vi "AP_2_launcher.vi"() -> ()   [LabVIEW 2023]
panel:
  in  "Cold head control launch":bool
  in  "Delay Control Launch":bool
  in  "Stop":bool
  in  "PDS Acquisition Launch Button":bool
  in  "PES Acquisition Launch Button":bool
  in  "Oscilloscope Launch Button":bool
  # "AP-2 Software Launcher"
  # "Welcome to the AP-2 software suite! Please seclect the software you wish to use."
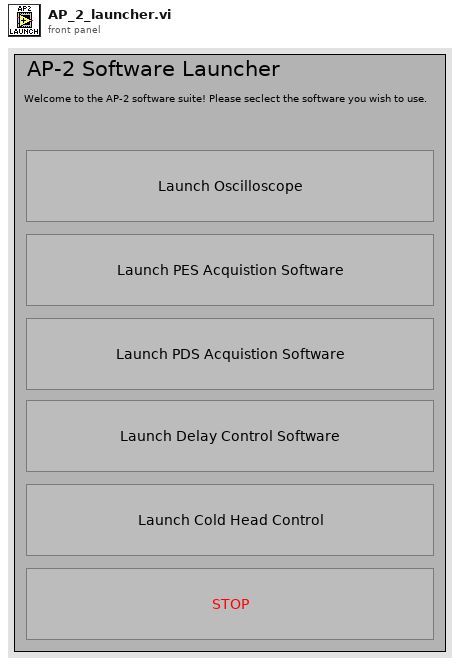
[diagram p1: front panel]
types:
  T1 = enum32{"Invalid", "Standard", "Closed", "Hidden", "Minimized", "Maximized"}
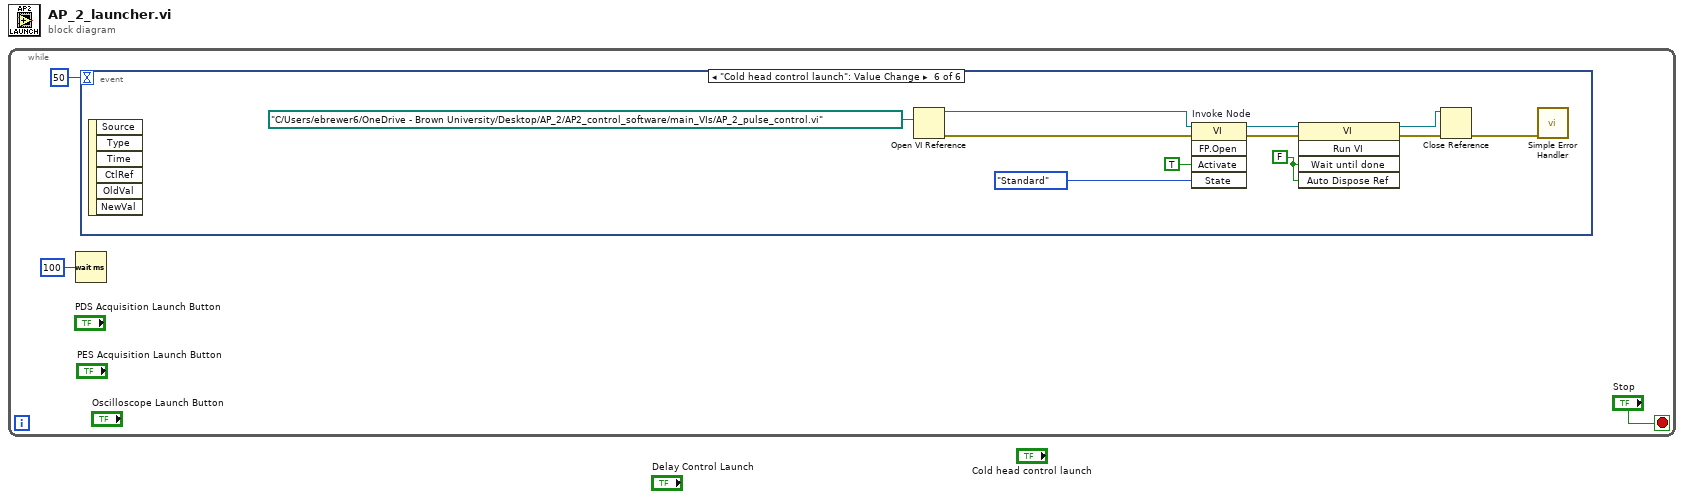
[diagram p0: block diagram]
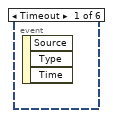
[diagram p2: hidden frame]
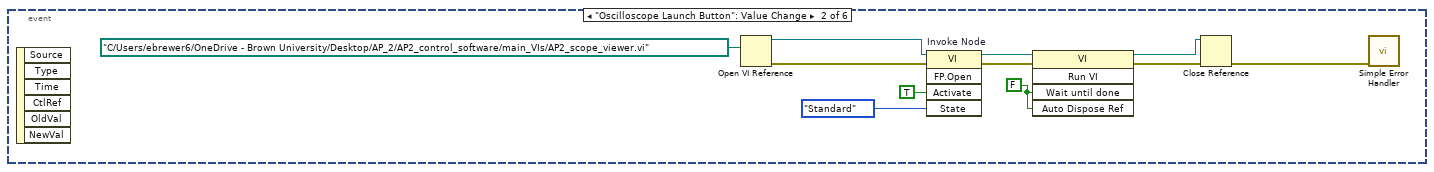
[diagram p3: hidden frame]
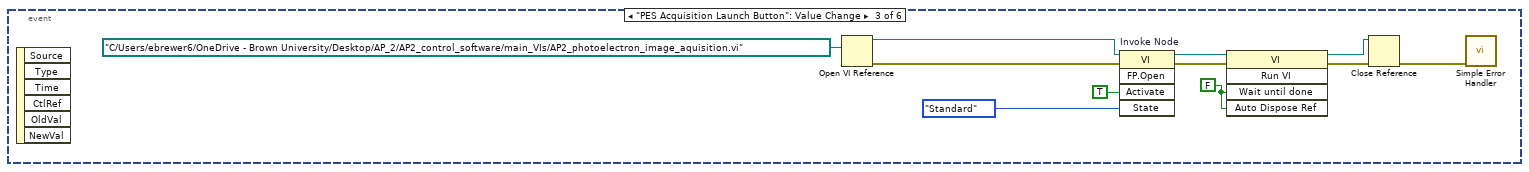
[diagram p4: hidden frame]
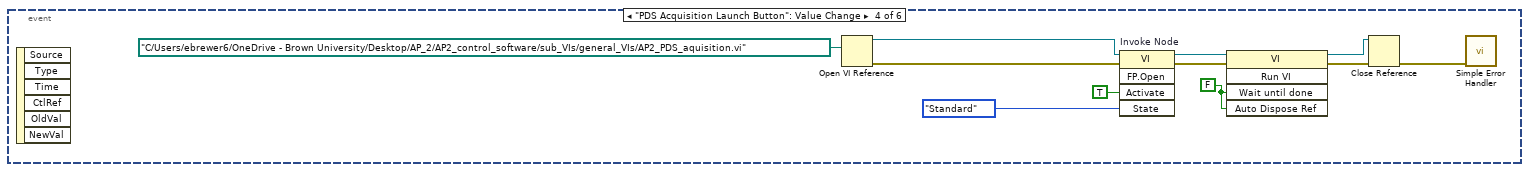
[diagram p5: hidden frame]
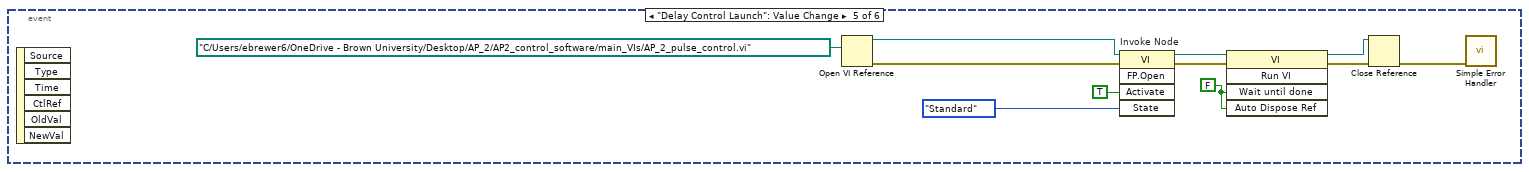
[diagram p6: hidden frame]
diagram:
  n1 = while {
    stop <- "Stop" stop-if-true
    n2 = Wait (ms)(milliseconds to wait=u32 100) -> ()  [unwired: 1 out]
    n3 = event shown="[5] \"Cold head control launch\": Value Change" {
      selector: _ -> [_ _ _ _ _ _]
      dyn-events: _ -> [_ _ _ _ _ _]
      timeout: 50 -> [_ _ _ _ _ _]
      event Timeout {
        n4 = event-data() -> ()  [unwired: 1 in, 3 out]
      }
      event "Oscilloscope Launch Button": Value Change {
        w7 = FALSE ("Wait Until Done")
        n5 = event-data() -> ()  [unwired: 1 in, 6 out]
        n6 = Open VI Reference(vi path=path "C:/Users/ebrewer6/OneDrive - Brown University/Desktop/AP_2/AP2_control_software/main_VIs/AP2_scope_viewer.vi") -> (vi reference=w8:refnum<vi>, error out=w9:errorcluster)  [unwired: 1 in, 4 out]
        n7 = invoke on="Invoke Node" class="VI" method="FP.Open"(reference=w8, error in=w9, "Activate"=TRUE ("Activate?"), "State"=T1."Standard") -> (reference out=w11:refnum<vi>, error out=w12:errorcluster)  [unwired: 1 in, 3 out]
        n8 = invoke class="VI" method="Run VI"(reference=w11, error in=w12, "Wait until done"=w7, "Auto Dispose Ref"=w7) -> (reference out=w13:refnum<vi>, error out=w14:errorcluster)  [unwired: 1 in, 3 out]
        n9 = Close Reference(reference=w13, error in (no error)=w14) -> (error out=w10:errorcluster)
        n10 = call <vilib>:"Simple Error Handler.vi"("error in (no error)"=w10) -> ()  [unwired: 1 in, 8 out]
      }
      event "PES Acquisition Launch Button": Value Change {
        w18 = FALSE ("Wait Until Done")
        n11 = event-data() -> ()  [unwired: 1 in, 6 out]
        n12 = Open VI Reference(vi path=path "C:/Users/ebrewer6/OneDrive - Brown University/Desktop/AP_2/AP2_control_software/main_VIs/AP2_photoelectron_image_aquisition.vi") -> (vi reference=w19:refnum<vi>, error out=w20:errorcluster)  [unwired: 1 in, 4 out]
        n13 = invoke on="Invoke Node" class="VI" method="FP.Open"(reference=w19, error in=w20, "Activate"=TRUE ("Activate?"), "State"=T1."Standard") -> (reference out=w22:refnum<vi>, error out=w23:errorcluster)  [unwired: 1 in, 3 out]
        n14 = invoke class="VI" method="Run VI"(reference=w22, error in=w23, "Wait until done"=w18, "Auto Dispose Ref"=w18) -> (reference out=w24:refnum<vi>, error out=w25:errorcluster)  [unwired: 1 in, 3 out]
        n15 = Close Reference(reference=w24, error in (no error)=w25) -> (error out=w21:errorcluster)
        n16 = call <vilib>:"Simple Error Handler.vi"("error in (no error)"=w21) -> ()  [unwired: 1 in, 8 out]
      }
      event "PDS Acquisition Launch Button": Value Change {
        w29 = FALSE ("Wait Until Done")
        n17 = event-data() -> ()  [unwired: 1 in, 6 out]
        n18 = Open VI Reference(vi path=path "C:/Users/ebrewer6/OneDrive - Brown University/Desktop/AP_2/AP2_control_software/sub_VIs/general_VIs/AP2_PDS_aquisition.vi") -> (vi reference=w30:refnum<vi>, error out=w31:errorcluster)  [unwired: 1 in, 4 out]
        n19 = invoke on="Invoke Node" class="VI" method="FP.Open"(reference=w30, error in=w31, "Activate"=TRUE ("Activate?"), "State"=T1."Standard") -> (reference out=w33:refnum<vi>, error out=w34:errorcluster)  [unwired: 1 in, 3 out]
        n20 = invoke class="VI" method="Run VI"(reference=w33, error in=w34, "Wait until done"=w29, "Auto Dispose Ref"=w29) -> (reference out=w35:refnum<vi>, error out=w36:errorcluster)  [unwired: 1 in, 3 out]
        n21 = Close Reference(reference=w35, error in (no error)=w36) -> (error out=w32:errorcluster)
        n22 = call <vilib>:"Simple Error Handler.vi"("error in (no error)"=w32) -> ()  [unwired: 1 in, 8 out]
      }
      event "Delay Control Launch": Value Change {
        w40 = FALSE ("Wait Until Done")
        n23 = event-data() -> ()  [unwired: 1 in, 6 out]
        n24 = Open VI Reference(vi path=path "C:/Users/ebrewer6/OneDrive - Brown University/Desktop/AP_2/AP2_control_software/main_VIs/AP_2_pulse_control.vi") -> (vi reference=w41:refnum<vi>, error out=w42:errorcluster)  [unwired: 1 in, 4 out]
        n25 = invoke on="Invoke Node" class="VI" method="FP.Open"(reference=w41, error in=w42, "Activate"=TRUE ("Activate?"), "State"=T1."Standard") -> (reference out=w44:refnum<vi>, error out=w45:errorcluster)  [unwired: 1 in, 3 out]
        n26 = invoke class="VI" method="Run VI"(reference=w44, error in=w45, "Wait until done"=w40, "Auto Dispose Ref"=w40) -> (reference out=w46:refnum<vi>, error out=w47:errorcluster)  [unwired: 1 in, 3 out]
        n27 = Close Reference(reference=w46, error in (no error)=w47) -> (error out=w43:errorcluster)
        n28 = call <vilib>:"Simple Error Handler.vi"("error in (no error)"=w43) -> ()  [unwired: 1 in, 8 out]
      }
      event "Cold head control launch": Value Change {
        w51 = FALSE ("Wait Until Done")
        n29 = event-data() -> ()  [unwired: 1 in, 6 out]
        n30 = Open VI Reference(vi path=path "C:/Users/ebrewer6/OneDrive - Brown University/Desktop/AP_2/AP2_control_software/main_VIs/AP_2_pulse_control.vi") -> (vi reference=w52:refnum<vi>, error out=w53:errorcluster)  [unwired: 1 in, 4 out]
        n31 = invoke on="Invoke Node" class="VI" method="FP.Open"(reference=w52, error in=w53, "Activate"=TRUE ("Activate?"), "State"=T1."Standard") -> (reference out=w55:refnum<vi>, error out=w56:errorcluster)  [unwired: 1 in, 3 out]
        n32 = invoke class="VI" method="Run VI"(reference=w55, error in=w56, "Wait until done"=w51, "Auto Dispose Ref"=w51) -> (reference out=w57:refnum<vi>, error out=w58:errorcluster)  [unwired: 1 in, 3 out]
        n33 = Close Reference(reference=w57, error in (no error)=w58) -> (error out=w54:errorcluster)
        n34 = call <vilib>:"Simple Error Handler.vi"("error in (no error)"=w54) -> ()  [unwired: 1 in, 8 out]
      }
    }
  }
